vi "Projet module.vi"() -> ()   [LabVIEW 2018]
panel:
  in  "?":bool
  out "ON":bool
  in  "Saisir l'identifiant de la carte":string
  out "La carte identifiée":picture
  in  "?":bool
  in  "STOP":bool
  # "Projet module : \nSystéme de réconnaissance des cartes étudiants\n\n \n                         Réalisée par:\n                      Yosra Massoud"
  # "Projet module \"Labview pour l'instrumentation\""
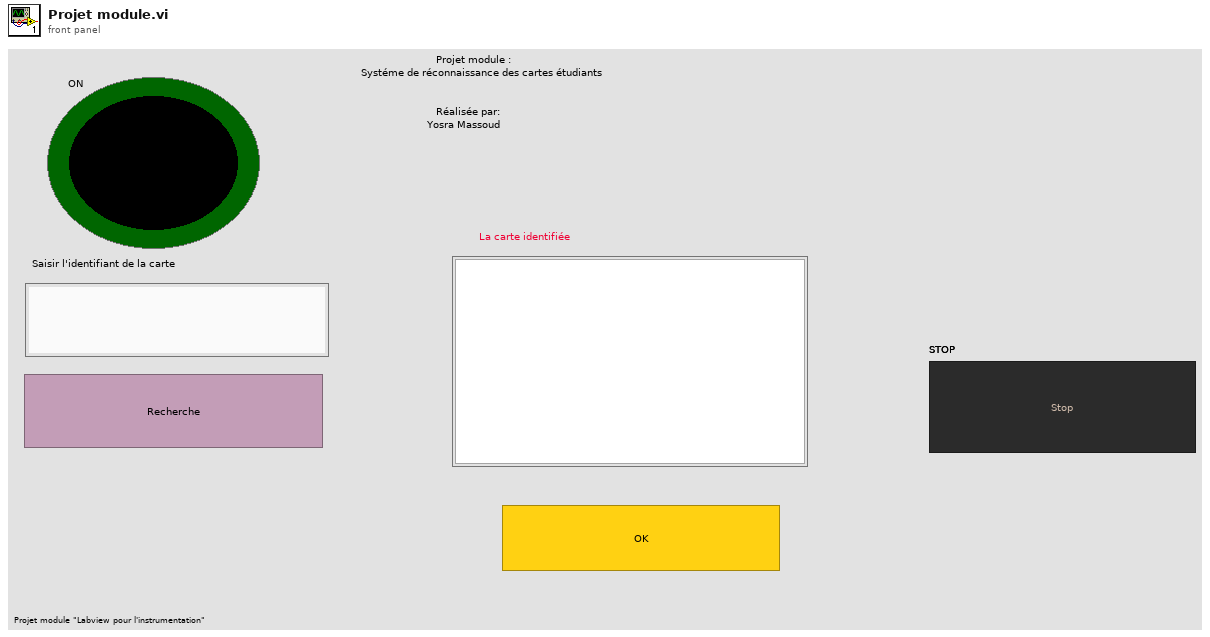
[diagram p1: front panel]
types:
  T1 = typedef "LVBoundsTypeDef.ctl" = cluster{"Width":u32, "Height":u32}
  T2 = typedef "imagedata.ctl" = cluster{"image type":i32, "image depth":i32, "image":u8[], "mask":u8[], "colors":u32[], "Rectangle":cluster{"left":i16, "top":i16, "right":i16, "bottom":i16}}
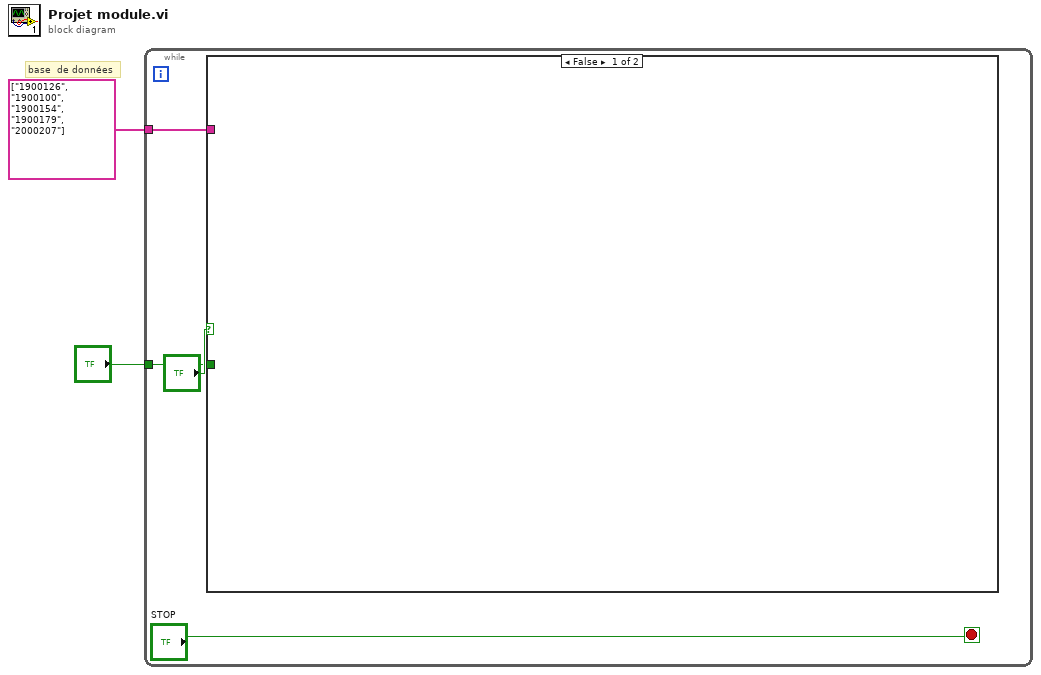
[diagram p0: block diagram]
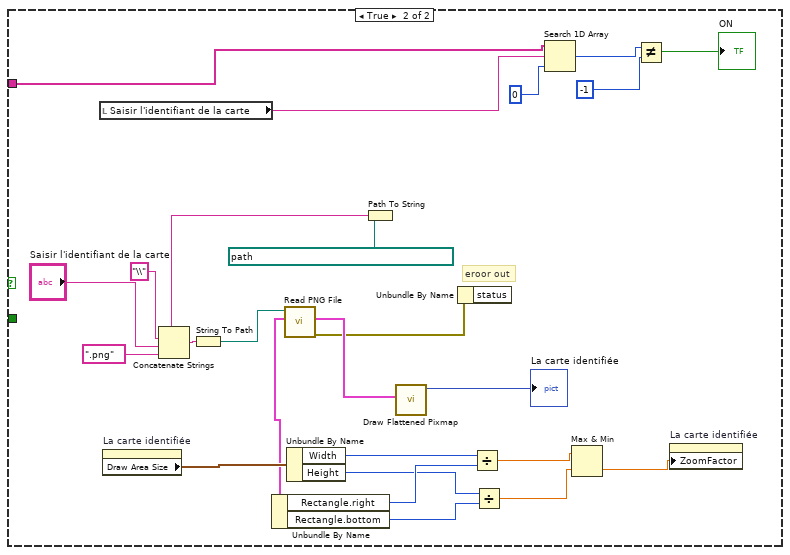
[diagram p2: hidden frame]
diagram:
  # "base  de données"
  n1 = while {
    tunnel: string[] ["1900126", "1900100", "1900154", "1900179", "2000207"] -> [w5]
    tunnel: "?" -> [w3]
    stop <- "STOP" stop-if-true
    n2 = case shown="False" "?" {
      tunnel: w5 -> [_ w8]
      tunnel: w3 -> [_ _]
      frame False {
      }
      frame True {
        # "eroor out"
        n3 = local read "Saisir l'identifiant de la carte"() -> (w13:string)
        n4 = property on="La carte identifiée" class="Pict"() -> ("Draw Area Size"=w29:T1)  [unwired: 2 in, 2 out]
        n5 = Unbundle By Name(w29) -> ("Width"=w27:u32, "Height"=w25:u32)
        n6 = Path To String(path=path "C:/Users/HP/Desktop/Base des données" ("path to JPEG file")) -> (string=w17:string)
        n7 = Concatenate Strings(w17, "\\", "Saisir l'identifiant de la carte", ".png") -> (w19:string)
        n8 = String To Path(string=w19) -> (path=w20:path)
        n9 = call <vilib>:"Read PNG File.vi"("path to PNG file"=w20) -> ("error out"=w7:errorcluster, "image data"=w28:T2)  [unwired: 8 in, 1 out]
        n10 = Unbundle By Name(w28) -> ("Rectangle.right"=w26:i16, "Rectangle.bottom"=w24:i16)
        n11 = call <vilib>:"Draw Flattened Pixmap.vi"("image data"=w28) -> ("new picture"=→"La carte identifiée":picture)  [unwired: 8 in]
        n12 = Unbundle By Name(w7) -> ()  [unwired: 1 out]
        n13 = Divide(x=w27, y=w26) -> (x/y=w23:dbl)
        n14 = Divide(x=w25, y=w24) -> (x/y=w22:dbl)
        n15 = Search 1D Array(1D array=w8, element=w13, start index (0)=0) -> (index of element=w12:i32)
        n16 = Max & Min(x=w23, y=w22) -> (min(x,y)=w21:dbl)  [unwired: 1 out]
        n17 = Not Equal?(x=w12, y=-1) -> (x != y?=→"ON":bool)
        n18 = property on="La carte identifiée" class="Pict"("ZoomFactor"=w21) -> ()  [unwired: 2 in, 2 out]
      }
    }
  }
